vi "Process triangle panel.vi"(1 "Panel triangle in":T1={"V0"=[], "V1"=[], "V2"=[], "E0"=[], "E1"=[], "E2"=[], "n^"=[], "Pc"=[], "Gamma'"=0.0, "V_transp."=0.0, "E0 link"=-1, "E1 link"=-1, "E2 link"=-1}) -> (0 "Panel triangle out":T1={"V0"=[], "V1"=[], "V2"=[], "E0"=[], "E1"=[], "E2"=[], "n^"=[], "Pc"=[], "Gamma'"=0.0, "V_transp."=0.0, "E0 link"=-1, "E1 link"=-1, "E2 link"=-1})   [LabVIEW 2017]
doc: "This VI must be run after any alteration to the triangles geometry involving scaling and rotation.\nThere is no need to run this VI after applying a translation."
uses:
  ctls/Triangle panel.ctl
  Dot product_3Dpf.vi
panel:
  # "PN 21/10/2017"
  # "Vertices"
  # "Edges"
  # "Unit normal"
  # "Control point"
  # "Edge\nlinks \n(tri index)"
  # "Vertices"
  # "Edges"
  # "Unit normal"
  # "Control point"
  # "Edge\nlinks \n(tri index)"
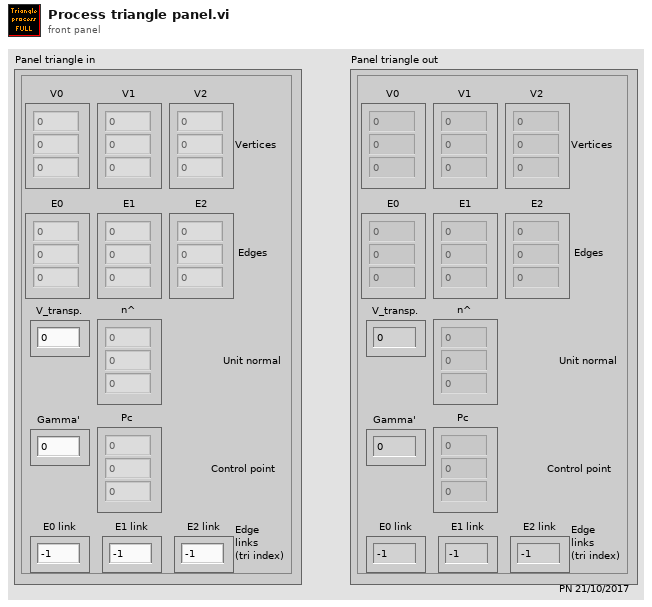
[diagram p1: front panel]
types:
  T1 = typedef "Triangle panel.ctl" = cluster{"V0":sgl[], "V1":sgl[], "V2":sgl[], "E0":sgl[], "E1":sgl[], "E2":sgl[], "n^":sgl[], "Pc":sgl[], "Gamma'":sgl, "V_transp.":sgl, "E0 link":i32, "E1 link":i32, "E2 link":i32}
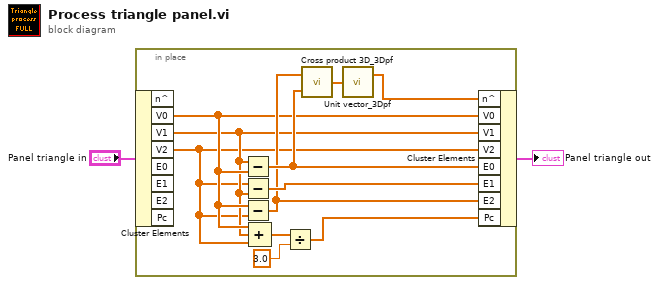
[diagram p0: block diagram]
diagram:
  n1 = in-place {
    n2 = in-place-cluster #1("Panel triangle in") -> ("V0"=w8:sgl[], "V1"=w7:sgl[], "V2"=w6:sgl[])  [unwired: 5 out]
    n3 = Subtract(x=w7, y=w8) -> (x-y=w11:sgl[])
    n4 = Subtract(x=w6, y=w7) -> (x-y=w10:sgl[])
    n5 = Subtract(x=w8, y=w6) -> (x-y=w9:sgl[])
    n6 = Compound Arithmetic op=ADD(w8, w7, w6) -> (w4:sgl[])
    n7 = Divide(x=w4, y=sgl 3.0) -> (x/y=w3:sgl[])
    n8 = call "Cross product 3D_3Dpf.vi"("B"=w11, "A"=w9) -> ("A x B"=w13:sgl[])
    n9 = call "Unit vector_3Dpf.vi"("Vector"=w13) -> ("Unit vector"=w12:sgl[])  [unwired: 1 out]
    n10 = in-place-cluster #1("n^"=w12, "V0"=w8, "V1"=w7, "V2"=w6, "E0"=w11, "E1"=w10, "E2"=w9, "Pc"=w3) -> (→"Panel triangle out":T1)
  }
